vi "Pickering 4 wire.vi"(4 "Ground config":T2={"X Channel Ground"="x12", "Y Channel Ground"="y1"}, 5 "Pickering status":path=path "C:/Local_LabVIEW/New Text Document.txt", 6 "configuration":T1={"Initialize"=FALSE, "Disconnect all?"=FALSE, "Discharge X channels?"=TRUE, "Discharge Y Channels?"=TRUE}, 7 "IVI Option String":string="Simulate=0,RangeCheck=1,QueryInstrStatus=0,Cache=1,DriverSetup=Model:40-726-511-M;", 8 "error in (no error)":errorcluster, 9 "Y Channels":string[][](array[combo])=[["NC", "NC"], ["y1", "NC"], ["y2", ""], ["y4", ""], ["NC", ""], ["y5", ""], ["y8", ""], ["y3", ""], ["NC", ""], ["y7", ""], ["y6", ""]], 10 "X Channels":string[](array[combo])=["x1", "x2", "x3", "x4", "x5", "x6", "x7", "x8", "x9", "x10", "x11"], 11 "VISA Resource Name":string="PXI13::13::INSTR") -> (0 "error out":errorcluster, 3 "instrument handle out":string)   [LabVIEW 2016, in "pickering.lvclass"]
uses:
  pickering.lvclass
  Typedefs/Channels-Array.ctl
  Typedefs/Channel-Cluster.ctl
  Typedefs/ChannelX-ComboBox.ctl
  Typedefs/ChannelY-ComboBox.ctl
panel:
  in  "Tab Control":enum32{"Crosspoint Selection", "Setup"}(tab)
  # "Lock-in 1: I+/I- -->AO0/AI0, board 0\n\nLock-in 3: V+/V-  --> AI0, board 1.  \n  V+/V- conencted to y3 and y4. OSC output should set the same as Lock-in 1\n\nLock-in 2: I2+/I2- -->AO1/AI1, board 0\n\nLock-in 4: V2+/V2- -> y7/y8"
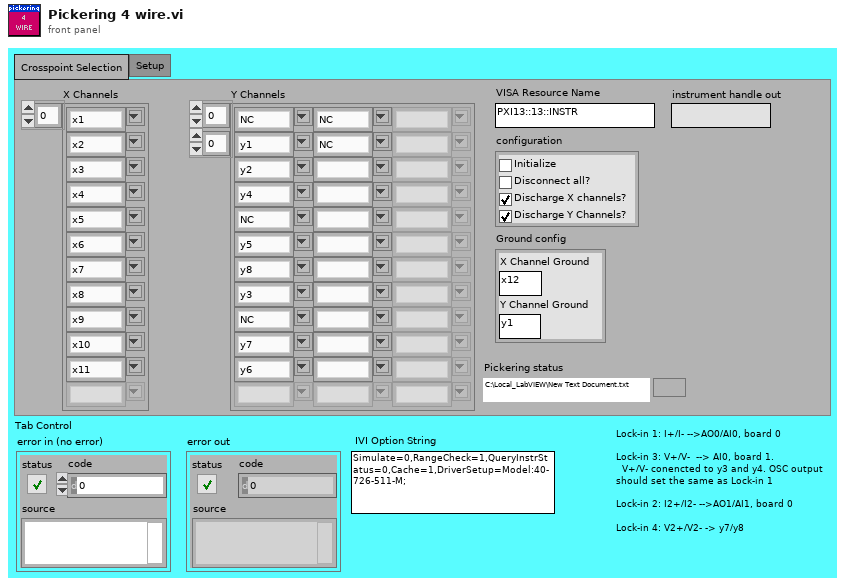
[diagram p1: front panel]
types:
  T1 = cluster{"Initialize":bool, "Disconnect all?":bool, "Discharge X channels?":bool, "Discharge Y Channels?":bool}
  T2 = cluster{"X Channel Ground":string, "Y Channel Ground":string}
  T3 = typedef "pickering.lvclass/Channels-Array.ctl" = T4[]
  T4 = typedef "pickering.lvclass/Channel-Cluster.ctl" = cluster{"Channel x":T5, "Channel y":T6}
  T5 = typedef "pickering.lvclass/ChannelX-ComboBox.ctl" = string
  T6 = typedef "pickering.lvclass/ChannelY-ComboBox.ctl" = string
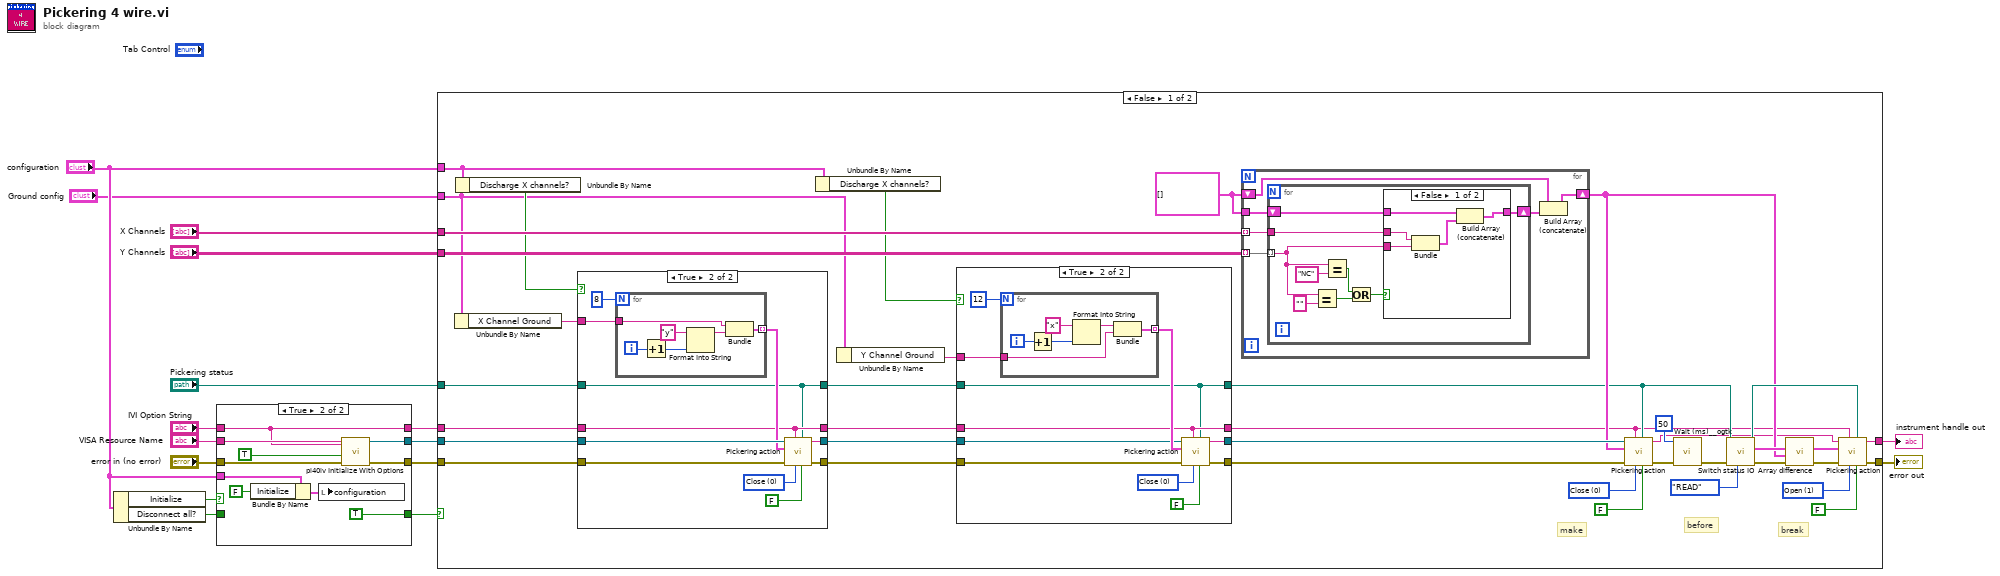
[diagram p0: block diagram]
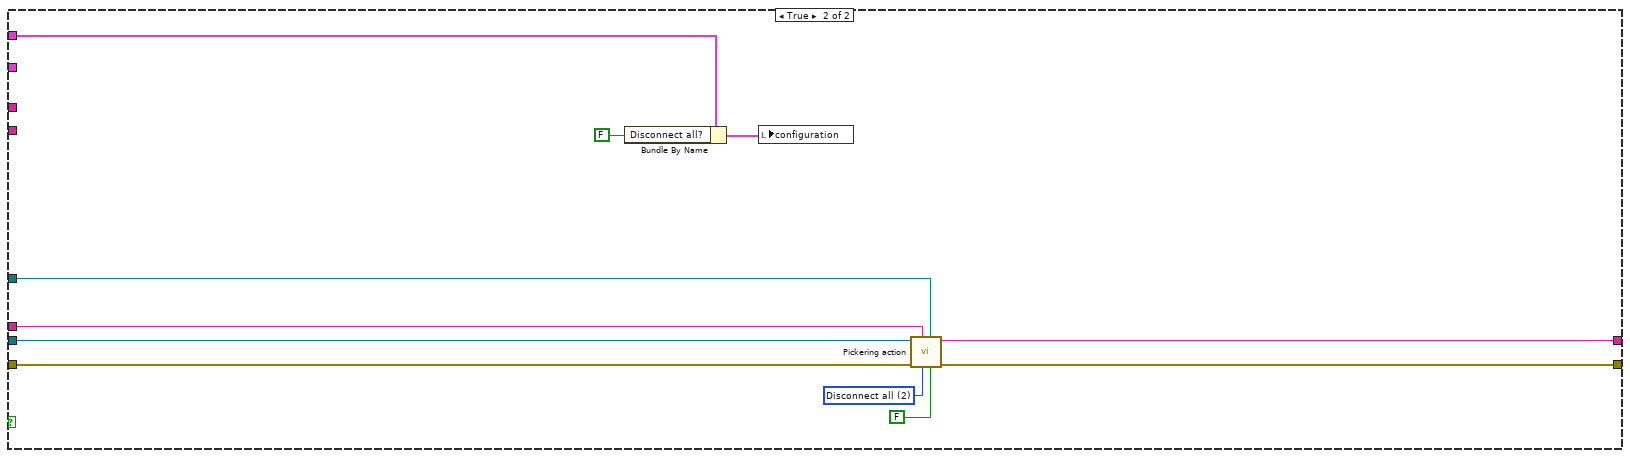
[diagram p5: hidden frame]
diagram:
  n1 = Unbundle By Name("configuration") -> ("Initialize"=w5:bool, "Disconnect all?"=w4:bool)
  n2 = case shown="True" w5 {
    tunnel: "VISA Resource Name" -> [w20 w30]
    tunnel: [w20 w27] -> w9
    tunnel: "IVI Option String" -> [w19 w29]
    tunnel: [w19 w29] -> w12
    tunnel: w4 -> [w18 _]
    tunnel: [w18 TRUE ("reset device")] -> w11
    tunnel: [w17 w26] -> w8
    tunnel: "error in (no error)" -> [w17 w24]
    tunnel: "configuration" -> [_ w21]
    frame False {
    }
    frame True {
      n3 = Bundle By Name(cluster=w21, "Initialize"=FALSE ("reset device")) -> (w23:T1)
      n4 = local write "configuration"(w23) -> ()
      n5 = call <instrlib>:"pi40iv Initialize With Options.vi"("option string"=w29, "error in (no error)"=w24, "reset device"=TRUE, "resource name"=w30) -> ("error out"=w26:errorcluster, "instrument handle out"=w27:refnum<k15>)  [unwired: 6 in]
    }
  }
  n6 = case shown="False" w11 {
    tunnel: "Y Channels" -> [w59 _]
    tunnel: "X Channels" -> [w56 _]
    tunnel: w12 -> [w68 w140]
    tunnel: w9 -> [w67 w142]
    tunnel: "Pickering status" -> [w66 w138]
    tunnel: w8 -> [w65 w141]
    tunnel: [w64 w136] -> w6
    tunnel: "configuration" -> [w37 w133]
    tunnel: [w35 w132] -> w2
    tunnel: "Ground config" -> [w31 _]
    frame False {
      w46 = u16 1 items=["Close", "Open", "Disconnect all"] ("Action")
      w53 = u16 0 items=["Close", "Open", "Disconnect all"] ("Action")
      w41 = T3 []
      # "break"
      # "before"
      # "make"
      n7 = Unbundle By Name(w31) -> ("X Channel Ground"=w33:string)
      n8 = Unbundle By Name(w37) -> ("Discharge X channels?"=w39:bool)
      n9 = case shown="True" w39 {
        tunnel: w33 -> [_ w83]
        tunnel: w68 -> [w70 w74]
        tunnel: w67 -> [w72 w81]
        tunnel: w66 -> [w69 w73]
        tunnel: w65 -> [w71 w77]
        tunnel: [w71 w76] -> w60
        tunnel: [w72 w75] -> w62
        tunnel: [w70 w74] -> w63
        tunnel: [w69 w73] -> w61
        frame False {
        }
        frame True {
          w78 = u16 0 items=["Close", "Open", "Disconnect all"] ("Action")
          n10 = for {
            N: 8 -> [_]
            tunnel: w83 -> [w85]
            tunnel: [w84] -> w80 mode=indexing
            i -> [w88]
            n11 = Increment(x=w88) -> (x+1=w87:i32)
            n12 = Format Into String(initial string="y", w87) -> (resulting string=w86:string)  [unwired: 2 in, 1 out]
            n13 = Bundle("X Channel Ground"=w85, w86) -> (w84:cluster{"X Channel Ground":string, string})  [unwired: 1 in]
          }
          n14 = call "Pickering action.vi"("Initialize"=FALSE, "Pickering status"=w73, "Action"=w78, "option string"=w74, "error in (no error)"=w77, "Channels Array"=w80, "instrument handle"=w81) -> ("error out"=w76:errorcluster, "instrument handle out"=w75:string)  [unwired: 3 in]
        }
      }
      n15 = Unbundle By Name(w37) -> ("Discharge X channels?"=w38:bool)
      n16 = Unbundle By Name(w31) -> ("Y Channel Ground"=w32:string)
      n17 = case shown="True" w38 {
        tunnel: w32 -> [_ w125]
        tunnel: w61 -> [w111 w115]
        tunnel: w62 -> [w113 w122]
        tunnel: w63 -> [w114 w118]
        tunnel: w60 -> [w112 w119]
        tunnel: [w114 w118] -> w34
        tunnel: [w112 w117] -> w57
        tunnel: [w113 w116] -> w58
        tunnel: [w111 w115] -> w40
        frame False {
        }
        frame True {
          w120 = u16 0 items=["Close", "Open", "Disconnect all"] ("Action")
          n18 = for {
            N: 12 -> [_]
            tunnel: w125 -> [w126]
            tunnel: [w128] -> w123 mode=indexing
            i -> [w130]
            n19 = Increment(x=w130) -> (x+1=w129:i32)
            n20 = Format Into String(initial string="x", w129) -> (resulting string=w127:string)  [unwired: 2 in, 1 out]
            n21 = Bundle(w127, "Y Channel Ground"=w126) -> (w128:cluster{string, "Y Channel Ground":string})  [unwired: 1 in]
          }
          n22 = call "Pickering action.vi"("Initialize"=FALSE, "Pickering status"=w115, "Action"=w120, "option string"=w118, "error in (no error)"=w119, "Channels Array"=w123, "instrument handle"=w122) -> ("error out"=w117:errorcluster, "instrument handle out"=w116:string)  [unwired: 3 in]
        }
      }
      n23 = for {
        tunnel: w59 -> [w94] mode=indexing
        tunnel: w56 -> [w95] mode=indexing
        shift-right: [w90] -> w42
        shift-left: w41 -> [w92]
        tunnel: w41 -> [w91]
        n24 = for {
          tunnel: w95 -> [w99]
          tunnel: w94 -> [w98] mode=indexing
          shift-right: [w97] -> w93
          shift-left: w91 -> [w96]
          n25 = Equal?(x=w98, y="") -> (x = y?=w101:bool)
          n26 = Equal?(x=w98, y="NC") -> (x = y?=w103:bool)
          n27 = Or(x=w103, y=w101) -> (x .or. y?=w102:bool)
          n28 = case shown="False" w102 {
            tunnel: w99 -> [w105 _]
            tunnel: w98 -> [w106 _]
            tunnel: [w108 w110] -> w97
            tunnel: w96 -> [w107 w110]
            frame False {
              n29 = Bundle("Channel x"=w105, "Channel y"=w106) -> (w109:cluster{"Channel x":string, "Channel y":string})  [unwired: 1 in]
              n30 = Build Array (concatenate)(w107, w109) -> (w108:T3)
            }
            frame True {
            }
          }
        }
        n31 = Build Array (concatenate)(w92, w93) -> (w90:T3)
      }
      n32 = call "Pickering action.vi"("Initialize"=FALSE, "Pickering status"=w40, "Action"=w53, "option string"=w34, "error in (no error)"=w57, "Channels Array"=w42, "instrument handle"=w58) -> ("error out"=w48:errorcluster, "instrument handle out"=w36:string)  [unwired: 3 in]
      n33 = call <userlib>:"Wait (ms)__ogtk.vi"("error in (no error)"=w48, "milliseconds to wait"=u32 50) -> ("error out"=w50:errorcluster)  [unwired: 8 in, 1 out]
      n34 = call "Switch status IO.vi"("mode"=enum16{"READ", "WRITE"}."READ", "error in (no error)"=w50, "Path"=w40) -> ("error out"=w44:errorcluster, "Channels out"=w49:T3, "Path out"=w47:path)  [unwired: 6 in]
      n35 = call "Array difference.vi"("error in (no error)"=w44, "Channels Array 2"=w42, "Channels Array"=w49) -> ("error out"=w45:errorcluster, "Array 1-(array1&2)"=w55:T3)  [unwired: 6 in, 1 out]
      n36 = call "Pickering action.vi"("Initialize"=FALSE, "Pickering status"=w47, "Action"=w46, "option string"=w34, "error in (no error)"=w45, "Channels Array"=w55, "instrument handle"=w36) -> ("error out"=w64:errorcluster, "instrument handle out"=w35:string)  [unwired: 3 in]
    }
    frame True {
      w139 = u16 2 items=["Close", "Open", "Disconnect all"] ("Action")
      n37 = Bundle By Name(cluster=w133, "Disconnect all?"=FALSE ("reset device")) -> (w134:T1)
      n38 = local write "configuration"(w134) -> ()
      n39 = call "Pickering action.vi"("Initialize"=FALSE, "Pickering status"=w138, "Action"=w139, "option string"=w140, "error in (no error)"=w141, "instrument handle"=w142) -> ("error out"=w136:errorcluster, "instrument handle out"=w132:string)  [unwired: 4 in]
    }
  }
  "error out" <- w6
  "instrument handle out" <- w2
